vi "TestGetValue.vi"(8 "error in (no error)":errorcluster) -> (0 "error out":errorcluster)   [LabVIEW 2019]
uses:
  <vilib>/addons/_JKI Toolkits/Caraya/classes/Assert/Assert Equal Value_Variant.vi
  <vilib>/addons/_JKI Toolkits/Caraya/classes/Test/Test.lvclass
  <vilib>/addons/_JKI Toolkits/Caraya/classes/Assert/Assert.lvclass
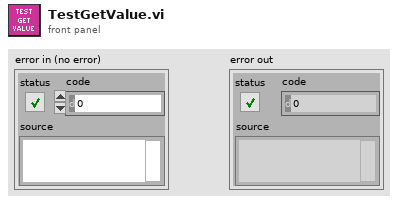
[diagram p1: front panel]
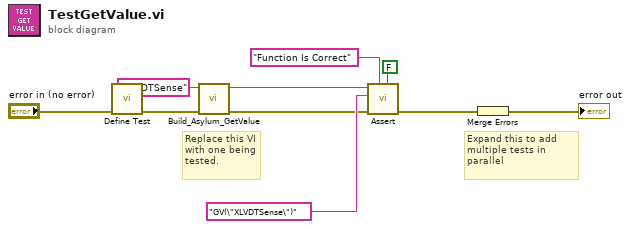
[diagram p0: block diagram]
diagram:
  # "Expand this to add multiple tests in parallel"
  # "Replace this VI with one being tested."
  n1 = call <vilib>:"Define Test.vi"("error in (no error)"="error in (no error)") -> ("error out"=w4:errorcluster)  [unwired: 10 in]
  n2 = call "Build_Asylum_GetValue.vi"("error in (no error)"=w4, "Value"="XLVDTSense") -> ("error out"=w3:errorcluster, "String"=w2:string)  [unwired: 8 in]
  n3 = call-poly <vilib>:"Assert.vi"("Assert Only? (F)"=FALSE, "Label"="Function Is Correct", "error in (no error)"=w3, "Y"="GV(\"XLVDTSense\")", "X"=w2) -> ("error out"=w8:errorcluster)  [unwired: 6 in]
  n4 = Merge Errors(w8) -> (→"error out":errorcluster)
